vi "Allocate Image Memory (Machine).vi"() -> (0 "error out":errorcluster, 2 "Process Memory":T1[](array[typedef]), 3 "Acquisition Memory":T1[](array[typedef]))   [LabVIEW 2018]
uses:
  <vilib>/vision/Image Controls.llb/IMAQ Image.ctl
  <vilib>/vision/NI_Vision_Development_Module.lvlib
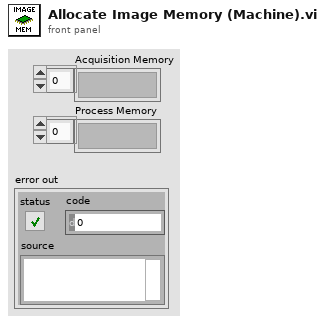
[diagram p1: front panel]
types:
  T1 = typedef "IMAQ Image.ctl" = refnum<image>
  T2 = typedef "IMAQ Circle" = cluster{"Center X":i32, "Center Y":i32, "Inner Radius":i32, "Outer Radius":i32, "Start Angle":dbl, "End Angle":dbl}
  T3 = typedef "Image Type" = u32
  T4 = typedef "ROI Descriptor" = cluster{"Global Rectangle":i32[], "Contours":cluster{"ID":enum32{"External", "Internal"}, "Type":u32, "Coordinates":i32[]}[]}
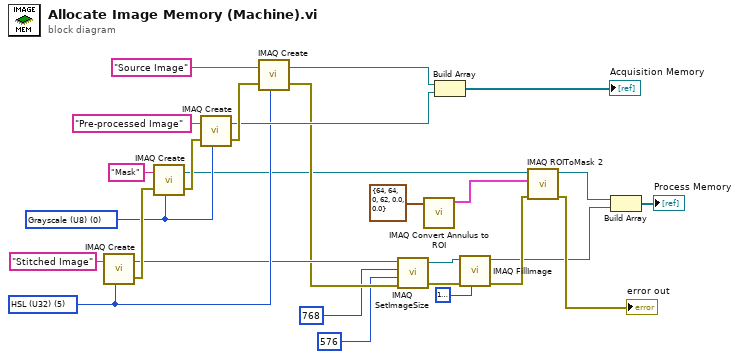
[diagram p0: block diagram]
diagram:
  w16 = T3 5 items=["Grayscale (U8)", "Grayscale (I16)", "Grayscale (SGL)", "Complex (CSG)", "RGB (U32)", "HSL (U32)", "RGB (U64)", "Grayscale (U16)"] ("Image Type")
  w22 = T3 0 items=["Grayscale (U8)", "Grayscale (I16)", "Grayscale (SGL)", "Complex (CSG)", "RGB (U32)", "HSL (U32)", "RGB (U64)", "Grayscale (U16)"] ("Image Type")
  n1 = call "IMAQ Create"("Image Name"="Stitched Image", "Image Type"=w16) -> ("New Image"=w15:T1, "error out"=w24:errorcluster)  [unwired: 3 in]
  n2 = call "IMAQ Create"("Image Name"="Mask", "Image Type"=w22, "error in (no error)"=w24) -> ("New Image"=w7:T1, "error out"=w23:errorcluster)  [unwired: 2 in]
  n3 = call "IMAQ Create"("Image Name"="Pre-processed Image", "Image Type"=w22, "error in (no error)"=w23) -> ("New Image"=w19:T1, "error out"=w20:errorcluster)  [unwired: 2 in]
  n4 = call "IMAQ Create"("Image Name"="Source Image", "Image Type"=w16, "error in (no error)"=w20) -> ("New Image"=w18:T1, "error out"=w14:errorcluster)  [unwired: 2 in]
  n5 = call "IMAQ SetImageSize"("error in (no error)"=w14, "Y Resolution"=576, "X Resolution"=768, "Image"=w15) -> ("error out"=w10:errorcluster, "Image Out"=w11:T1)  [unwired: 1 in]
  n6 = call "IMAQ Convert Annulus to ROI"("Annulus"=T2 {"Center X"=64, "Center Y"=64, "Inner Radius"=0, "Outer Radius"=62, "Start Angle"=0.0, "End Angle"=0.0}) -> ("ROI Descriptor"=w8:T4)  [unwired: 8 in, 1 out]
  n7 = Build Array(w18, w19) -> (→"Acquisition Memory":T1[])
  n8 = call "IMAQ FillImage"("Color Pixel Value"=u32 16777216, "error in (no error)"=w10, "Image"=w11) -> ("error out"=w6:errorcluster, "Image Out"=w4:T1)  [unwired: 7 in]
  n9 = call "IMAQ ROIToMask 2"("error in (no error)"=w6, "ROI Descriptor"=w8, "Image"=w7) -> ("error out"=→"error out":errorcluster, "Image Out"=w3:T1)  [unwired: 6 in, 1 out]
  n10 = Build Array(w3, w4) -> (→"Process Memory":T1[])
